vi "PCO_General.vi"() -> (0 "PCO_General":T1 {"PCO_CameraType"."wCamType" format="%x"; "PCO_CameraType"."wCamSubType" format="%x"; "PCO_CameraType"."InterfaceType" format="%x"; "dwCamHealthWarnings" format="%x"; "dwCamHealthErrors" format="%x"; "dwCamHealthStatus" format="%x"}, 1 "PCO_General_Raw":T2, 2 "Length":u16, 3 "Raw_Length":u16)   [LabVIEW 2019, in "SDK.lvlib" / "Structures.lvlib"]
doc: "Use this template to build a VI to use as a subVI."
uses:
  Structures.lvlib
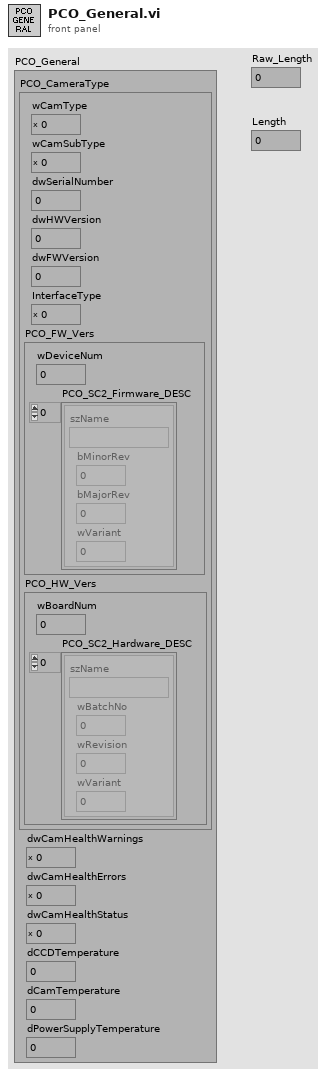
[diagram p1: front panel]
types:
  T1 = cluster{"PCO_CameraType":cluster{"wCamType":u16, "wCamSubType":u16, "dwSerialNumber":u32, "dwHWVersion":u32, "dwFWVersion":u32, "InterfaceType":u16, "PCO_FW_Vers":cluster{"wDeviceNum":u16, "PCO_SC2_Firmware_DESC":cluster{"szName":string, "bMinorRev":u8, "bMajorRev":u8, "wVariant":u16}[]}, "PCO_HW_Vers":cluster{"wBoardNum":u16, "PCO_SC2_Hardware_DESC":cluster{"szName":string, "wBatchNo":u16, "wRevision":u16, "wVariant":u16}[]}}, "dwCamHealthWarnings":u32, "dwCamHealthErrors":u32, "dwCamHealthStatus":u32, "dCCDTemperature":dbl, "dCamTemperature":dbl, "dPowerSupplyTemperature":dbl}
  T2 = cluster{"wSize":u16, "ZZwAlignDummy1":u16, "PCO_CameraType_Raw":cluster{"wSize":u16, "wCamType":u16, "wCamSubType":u16, "zzwAlignDummy1":u16, "dwSerialNumber":u32, "dwHWVersion":u32, "dwFWVersion":u32, "wInterfaceType":u16, "PCO_FW_Vers_Raw":cluster{"wDeviceNum":u16, "PCO_SC2_Firmware_DESC":cluster{"PCO_SC2_FW_Desc_Raw":cluster{"szName":cluster{u8, u8, u8, u8, u8, u8, u8, u8, u8, u8, u8, u8, u8, u8, u8, u8}, "bMinorRev":u8, "bMajorRev":u8, "wVariant":u16, "zzwDummy":cluster{u16, u16, u16, u16, u16, u16, u16, u16, u16, u16, u16, u16, u16, u16, u16, u16, u16, u16, u16, u16, u16, u16}}, "PCO_SC2_FW_Desc_Raw":cluster{"szName":cluster{u8, u8, u8, u8, u8, u8, u8, u8, u8, u8, u8, u8, u8, u8, u8, u8}, "bMinorRev":u8, "bMajorRev":u8, "wVariant":u16, "zzwDummy":cluster{u16, u16, u16, u16, u16, u16, u16, u16, u16, u16, u16, u16, u16, u16, u16, u16, u16, u16, u16, u16, u16, u16}}, "PCO_SC2_FW_Desc_Raw":cluster{"szName":cluster{u8, u8, u8, u8, u8, u8, u8, u8, u8, u8, u8, u8, u8, u8, u8, u8}, "bMinorRev":u8, "bMajorRev":u8, "wVariant":u16, "zzwDummy":cluster{u16, u16, u16, u16, u16, u16, u16, u16, u16, u16, u16, u16, u16, u16, u16, u16, u16, u16, u16, u16, u16, u16}}, "PCO_SC2_FW_Desc_Raw":cluster{"szName":cluster{u8, u8, u8, u8, u8, u8, u8, u8, u8, u8, u8, u8, u8, u8, u8, u8}, "bMinorRev":u8, "bMajorRev":u8, "wVariant":u16, "zzwDummy":cluster{u16, u16, u16, u16, u16, u16, u16, u16, u16, u16, u16, u16, u16, u16, u16, u16, u16, u16, u16, u16, u16, u16}}, "PCO_SC2_FW_Desc_Raw":cluster{"szName":cluster{u8, u8, u8, u8, u8, u8, u8, u8, u8, u8, u8, u8, u8, u8, u8, u8}, "bMinorRev":u8, "bMajorRev":u8, "wVariant":u16, "zzwDummy":cluster{u16, u16, u16, u16, u16, u16, u16, u16, u16, u16, u16, u16, u16, u16, u16, u16, u16, u16, u16, u16, u16, u16}}, "PCO_SC2_FW_Desc_Raw":cluster{"szName":cluster{u8, u8, u8, u8, u8, u8, u8, u8, u8, u8, u8, u8, u8, u8, u8, u8}, "bMinorRev":u8, "bMajorRev":u8, "wVariant":u16, "zzwDummy":cluster{u16, u16, u16, u16, u16, u16, u16, u16, u16, u16, u16, u16, u16, u16, u16, u16, u16, u16, u16, u16, u16, u16}}, "PCO_SC2_FW_Desc_Raw":cluster{"szName":cluster{u8, u8, u8, u8, u8, u8, u8, u8, u8, u8, u8, u8, u8, u8, u8, u8}, "bMinorRev":u8, "bMajorRev":u8, "wVariant":u16, "zzwDummy":cluster{u16, u16, u16, u16, u16, u16, u16, u16, u16, u16, u16, u16, u16, u16, u16, u16, u16, u16, u16, u16, u16, u16}}, "PCO_SC2_FW_Desc_Raw":cluster{"szName":cluster{u8, u8, u8, u8, u8, u8, u8, u8, u8, u8, u8, u8, u8, u8, u8, u8}, "bMinorRev":u8, "bMajorRev":u8, "wVariant":u16, "zzwDummy":cluster{u16, u16, u16, u16, u16, u16, u16, u16, u16, u16, u16, u16, u16, u16, u16, u16, u16, u16, u16, u16, u16, u16}}, "PCO_SC2_FW_Desc_Raw":cluster{"szName":cluster{u8, u8, u8, u8, u8, u8, u8, u8, u8, u8, u8, u8, u8, u8, u8, u8}, "bMinorRev":u8, "bMajorRev":u8, "wVariant":u16, "zzwDummy":cluster{u16, u16, u16, u16, u16, u16, u16, u16, u16, u16, u16, u16, u16, u16, u16, u16, u16, u16, u16, u16, u16, u16}}, "PCO_SC2_FW_Desc_Raw":cluster{"szName":cluster{u8, u8, u8, u8, u8, u8, u8, u8, u8, u8, u8, u8, u8, u8, u8, u8}, "bMinorRev":u8, "bMajorRev":u8, "wVariant":u16, "zzwDummy":cluster{u16, u16, u16, u16, u16, u16, u16, u16, u16, u16, u16, u16, u16, u16, u16, u16, u16, u16, u16, u16, u16, u16}}}}, "PCO_HW_Vers_Raw":cluster{"wBoardNum":u16, "PCO_SC2_Hardware_DESC":cluster{"PCO_SC2_HW_Desc_Raw":cluster{"szName":cluster{u8, u8, u8, u8, u8, u8, u8, u8, u8, u8, u8, u8, u8, u8, u8, u8}, "wBatchNo":u16, "wRevision":u16, "wVariant":u16, "zzwDummy":cluster{u16, u16, u16, u16, u16, u16, u16, u16, u16, u16, u16, u16, u16, u16, u16, u16, u16, u16, u16, u16}}, "PCO_SC2_HW_Desc_Raw":cluster{"szName":cluster{u8, u8, u8, u8, u8, u8, u8, u8, u8, u8, u8, u8, u8, u8, u8, u8}, "wBatchNo":u16, "wRevision":u16, "wVariant":u16, "zzwDummy":cluster{u16, u16, u16, u16, u16, u16, u16, u16, u16, u16, u16, u16, u16, u16, u16, u16, u16, u16, u16, u16}}, "PCO_SC2_HW_Desc_Raw":cluster{"szName":cluster{u8, u8, u8, u8, u8, u8, u8, u8, u8, u8, u8, u8, u8, u8, u8, u8}, "wBatchNo":u16, "wRevision":u16, "wVariant":u16, "zzwDummy":cluster{u16, u16, u16, u16, u16, u16, u16, u16, u16, u16, u16, u16, u16, u16, u16, u16, u16, u16, u16, u16}}, "PCO_SC2_HW_Desc_Raw":cluster{"szName":cluster{u8, u8, u8, u8, u8, u8, u8, u8, u8, u8, u8, u8, u8, u8, u8, u8}, "wBatchNo":u16, "wRevision":u16, "wVariant":u16, "zzwDummy":cluster{u16, u16, u16, u16, u16, u16, u16, u16, u16, u16, u16, u16, u16, u16, u16, u16, u16, u16, u16, u16}}, "PCO_SC2_HW_Desc_Raw":cluster{"szName":cluster{u8, u8, u8, u8, u8, u8, u8, u8, u8, u8, u8, u8, u8, u8, u8, u8}, "wBatchNo":u16, "wRevision":u16, "wVariant":u16, "zzwDummy":cluster{u16, u16, u16, u16, u16, u16, u16, u16, u16, u16, u16, u16, u16, u16, u16, u16, u16, u16, u16, u16}}, "PCO_SC2_HW_Desc_Raw":cluster{"szName":cluster{u8, u8, u8, u8, u8, u8, u8, u8, u8, u8, u8, u8, u8, u8, u8, u8}, "wBatchNo":u16, "wRevision":u16, "wVariant":u16, "zzwDummy":cluster{u16, u16, u16, u16, u16, u16, u16, u16, u16, u16, u16, u16, u16, u16, u16, u16, u16, u16, u16, u16}}, "PCO_SC2_HW_Desc_Raw":cluster{"szName":cluster{u8, u8, u8, u8, u8, u8, u8, u8, u8, u8, u8, u8, u8, u8, u8, u8}, "wBatchNo":u16, "wRevision":u16, "wVariant":u16, "zzwDummy":cluster{u16, u16, u16, u16, u16, u16, u16, u16, u16, u16, u16, u16, u16, u16, u16, u16, u16, u16, u16, u16}}, "PCO_SC2_HW_Desc_Raw":cluster{"szName":cluster{u8, u8, u8, u8, u8, u8, u8, u8, u8, u8, u8, u8, u8, u8, u8, u8}, "wBatchNo":u16, "wRevision":u16, "wVariant":u16, "zzwDummy":cluster{u16, u16, u16, u16, u16, u16, u16, u16, u16, u16, u16, u16, u16, u16, u16, u16, u16, u16, u16, u16}}, "PCO_SC2_HW_Desc_Raw":cluster{"szName":cluster{u8, u8, u8, u8, u8, u8, u8, u8, u8, u8, u8, u8, u8, u8, u8, u8}, "wBatchNo":u16, "wRevision":u16, "wVariant":u16, "zzwDummy":cluster{u16, u16, u16, u16, u16, u16, u16, u16, u16, u16, u16, u16, u16, u16, u16, u16, u16, u16, u16, u16}}, "PCO_SC2_HW_Desc_Raw":cluster{"szName":cluster{u8, u8, u8, u8, u8, u8, u8, u8, u8, u8, u8, u8, u8, u8, u8, u8}, "wBatchNo":u16, "wRevision":u16, "wVariant":u16, "zzwDummy":cluster{u16, u16, u16, u16, u16, u16, u16, u16, u16, u16, u16, u16, u16, u16, u16, u16, u16, u16, u16, u16}}}}, "zzWDummy":cluster{u16, u16, u16, u16, u16, u16, u16, u16, u16, u16, u16, u16, u16, u16, u16, u16, u16, u16, u16, u16, u16, u16, u16, u16, u16, u16, u16, u16, u16, u16, u16, u16, u16, u16, u16, u16, u16, u16, u16}}, "dwCamHealthWarnings":u32, "dwCamHealthErrors":u32, "dwCamHealthStatus":u32, "sCCDTemperature":i16, "sCamTemperature":i16, "sPowerSupplyTemperature":i16, "ZZwDummy":cluster{u16, u16, u16, u16, u16, u16, u16, u16, u16, u16, u16, u16, u16, u16, u16, u16, u16, u16, u16, u16, u16, u16, u16, u16, u16, u16, u16, u16, u16, u16, u16, u16, u16, u16, u16, u16, u16}}
  T3 = cluster{u16, u16, u16, u16, u16, u16, u16, u16, u16, u16, u16, u16, u16, u16, u16, u16, u16, u16, u16, u16, u16, u16, u16, u16, u16, u16, u16, u16, u16, u16, u16, u16, u16, u16, u16, u16, u16}
  T4 = cluster{"wCamType":u16, "wCamSubType":u16, "dwSerialNumber":u32, "dwHWVersion":u32, "dwFWVersion":u32, "InterfaceType":u16, "PCO_FW_Vers":cluster{"wDeviceNum":u16, "PCO_SC2_Firmware_DESC":cluster{"szName":string, "bMinorRev":u8, "bMajorRev":u8, "wVariant":u16}[]}, "PCO_HW_Vers":cluster{"wBoardNum":u16, "PCO_SC2_Hardware_DESC":cluster{"szName":string, "wBatchNo":u16, "wRevision":u16, "wVariant":u16}[]}}
  T5 = cluster{"wSize":u16, "wCamType":u16, "wCamSubType":u16, "zzwAlignDummy1":u16, "dwSerialNumber":u32, "dwHWVersion":u32, "dwFWVersion":u32, "wInterfaceType":u16, "PCO_FW_Vers_Raw":cluster{"wDeviceNum":u16, "PCO_SC2_Firmware_DESC":cluster{"PCO_SC2_FW_Desc_Raw":cluster{"szName":cluster{u8, u8, u8, u8, u8, u8, u8, u8, u8, u8, u8, u8, u8, u8, u8, u8}, "bMinorRev":u8, "bMajorRev":u8, "wVariant":u16, "zzwDummy":cluster{u16, u16, u16, u16, u16, u16, u16, u16, u16, u16, u16, u16, u16, u16, u16, u16, u16, u16, u16, u16, u16, u16}}, "PCO_SC2_FW_Desc_Raw":cluster{"szName":cluster{u8, u8, u8, u8, u8, u8, u8, u8, u8, u8, u8, u8, u8, u8, u8, u8}, "bMinorRev":u8, "bMajorRev":u8, "wVariant":u16, "zzwDummy":cluster{u16, u16, u16, u16, u16, u16, u16, u16, u16, u16, u16, u16, u16, u16, u16, u16, u16, u16, u16, u16, u16, u16}}, "PCO_SC2_FW_Desc_Raw":cluster{"szName":cluster{u8, u8, u8, u8, u8, u8, u8, u8, u8, u8, u8, u8, u8, u8, u8, u8}, "bMinorRev":u8, "bMajorRev":u8, "wVariant":u16, "zzwDummy":cluster{u16, u16, u16, u16, u16, u16, u16, u16, u16, u16, u16, u16, u16, u16, u16, u16, u16, u16, u16, u16, u16, u16}}, "PCO_SC2_FW_Desc_Raw":cluster{"szName":cluster{u8, u8, u8, u8, u8, u8, u8, u8, u8, u8, u8, u8, u8, u8, u8, u8}, "bMinorRev":u8, "bMajorRev":u8, "wVariant":u16, "zzwDummy":cluster{u16, u16, u16, u16, u16, u16, u16, u16, u16, u16, u16, u16, u16, u16, u16, u16, u16, u16, u16, u16, u16, u16}}, "PCO_SC2_FW_Desc_Raw":cluster{"szName":cluster{u8, u8, u8, u8, u8, u8, u8, u8, u8, u8, u8, u8, u8, u8, u8, u8}, "bMinorRev":u8, "bMajorRev":u8, "wVariant":u16, "zzwDummy":cluster{u16, u16, u16, u16, u16, u16, u16, u16, u16, u16, u16, u16, u16, u16, u16, u16, u16, u16, u16, u16, u16, u16}}, "PCO_SC2_FW_Desc_Raw":cluster{"szName":cluster{u8, u8, u8, u8, u8, u8, u8, u8, u8, u8, u8, u8, u8, u8, u8, u8}, "bMinorRev":u8, "bMajorRev":u8, "wVariant":u16, "zzwDummy":cluster{u16, u16, u16, u16, u16, u16, u16, u16, u16, u16, u16, u16, u16, u16, u16, u16, u16, u16, u16, u16, u16, u16}}, "PCO_SC2_FW_Desc_Raw":cluster{"szName":cluster{u8, u8, u8, u8, u8, u8, u8, u8, u8, u8, u8, u8, u8, u8, u8, u8}, "bMinorRev":u8, "bMajorRev":u8, "wVariant":u16, "zzwDummy":cluster{u16, u16, u16, u16, u16, u16, u16, u16, u16, u16, u16, u16, u16, u16, u16, u16, u16, u16, u16, u16, u16, u16}}, "PCO_SC2_FW_Desc_Raw":cluster{"szName":cluster{u8, u8, u8, u8, u8, u8, u8, u8, u8, u8, u8, u8, u8, u8, u8, u8}, "bMinorRev":u8, "bMajorRev":u8, "wVariant":u16, "zzwDummy":cluster{u16, u16, u16, u16, u16, u16, u16, u16, u16, u16, u16, u16, u16, u16, u16, u16, u16, u16, u16, u16, u16, u16}}, "PCO_SC2_FW_Desc_Raw":cluster{"szName":cluster{u8, u8, u8, u8, u8, u8, u8, u8, u8, u8, u8, u8, u8, u8, u8, u8}, "bMinorRev":u8, "bMajorRev":u8, "wVariant":u16, "zzwDummy":cluster{u16, u16, u16, u16, u16, u16, u16, u16, u16, u16, u16, u16, u16, u16, u16, u16, u16, u16, u16, u16, u16, u16}}, "PCO_SC2_FW_Desc_Raw":cluster{"szName":cluster{u8, u8, u8, u8, u8, u8, u8, u8, u8, u8, u8, u8, u8, u8, u8, u8}, "bMinorRev":u8, "bMajorRev":u8, "wVariant":u16, "zzwDummy":cluster{u16, u16, u16, u16, u16, u16, u16, u16, u16, u16, u16, u16, u16, u16, u16, u16, u16, u16, u16, u16, u16, u16}}}}, "PCO_HW_Vers_Raw":cluster{"wBoardNum":u16, "PCO_SC2_Hardware_DESC":cluster{"PCO_SC2_HW_Desc_Raw":cluster{"szName":cluster{u8, u8, u8, u8, u8, u8, u8, u8, u8, u8, u8, u8, u8, u8, u8, u8}, "wBatchNo":u16, "wRevision":u16, "wVariant":u16, "zzwDummy":cluster{u16, u16, u16, u16, u16, u16, u16, u16, u16, u16, u16, u16, u16, u16, u16, u16, u16, u16, u16, u16}}, "PCO_SC2_HW_Desc_Raw":cluster{"szName":cluster{u8, u8, u8, u8, u8, u8, u8, u8, u8, u8, u8, u8, u8, u8, u8, u8}, "wBatchNo":u16, "wRevision":u16, "wVariant":u16, "zzwDummy":cluster{u16, u16, u16, u16, u16, u16, u16, u16, u16, u16, u16, u16, u16, u16, u16, u16, u16, u16, u16, u16}}, "PCO_SC2_HW_Desc_Raw":cluster{"szName":cluster{u8, u8, u8, u8, u8, u8, u8, u8, u8, u8, u8, u8, u8, u8, u8, u8}, "wBatchNo":u16, "wRevision":u16, "wVariant":u16, "zzwDummy":cluster{u16, u16, u16, u16, u16, u16, u16, u16, u16, u16, u16, u16, u16, u16, u16, u16, u16, u16, u16, u16}}, "PCO_SC2_HW_Desc_Raw":cluster{"szName":cluster{u8, u8, u8, u8, u8, u8, u8, u8, u8, u8, u8, u8, u8, u8, u8, u8}, "wBatchNo":u16, "wRevision":u16, "wVariant":u16, "zzwDummy":cluster{u16, u16, u16, u16, u16, u16, u16, u16, u16, u16, u16, u16, u16, u16, u16, u16, u16, u16, u16, u16}}, "PCO_SC2_HW_Desc_Raw":cluster{"szName":cluster{u8, u8, u8, u8, u8, u8, u8, u8, u8, u8, u8, u8, u8, u8, u8, u8}, "wBatchNo":u16, "wRevision":u16, "wVariant":u16, "zzwDummy":cluster{u16, u16, u16, u16, u16, u16, u16, u16, u16, u16, u16, u16, u16, u16, u16, u16, u16, u16, u16, u16}}, "PCO_SC2_HW_Desc_Raw":cluster{"szName":cluster{u8, u8, u8, u8, u8, u8, u8, u8, u8, u8, u8, u8, u8, u8, u8, u8}, "wBatchNo":u16, "wRevision":u16, "wVariant":u16, "zzwDummy":cluster{u16, u16, u16, u16, u16, u16, u16, u16, u16, u16, u16, u16, u16, u16, u16, u16, u16, u16, u16, u16}}, "PCO_SC2_HW_Desc_Raw":cluster{"szName":cluster{u8, u8, u8, u8, u8, u8, u8, u8, u8, u8, u8, u8, u8, u8, u8, u8}, "wBatchNo":u16, "wRevision":u16, "wVariant":u16, "zzwDummy":cluster{u16, u16, u16, u16, u16, u16, u16, u16, u16, u16, u16, u16, u16, u16, u16, u16, u16, u16, u16, u16}}, "PCO_SC2_HW_Desc_Raw":cluster{"szName":cluster{u8, u8, u8, u8, u8, u8, u8, u8, u8, u8, u8, u8, u8, u8, u8, u8}, "wBatchNo":u16, "wRevision":u16, "wVariant":u16, "zzwDummy":cluster{u16, u16, u16, u16, u16, u16, u16, u16, u16, u16, u16, u16, u16, u16, u16, u16, u16, u16, u16, u16}}, "PCO_SC2_HW_Desc_Raw":cluster{"szName":cluster{u8, u8, u8, u8, u8, u8, u8, u8, u8, u8, u8, u8, u8, u8, u8, u8}, "wBatchNo":u16, "wRevision":u16, "wVariant":u16, "zzwDummy":cluster{u16, u16, u16, u16, u16, u16, u16, u16, u16, u16, u16, u16, u16, u16, u16, u16, u16, u16, u16, u16}}, "PCO_SC2_HW_Desc_Raw":cluster{"szName":cluster{u8, u8, u8, u8, u8, u8, u8, u8, u8, u8, u8, u8, u8, u8, u8, u8}, "wBatchNo":u16, "wRevision":u16, "wVariant":u16, "zzwDummy":cluster{u16, u16, u16, u16, u16, u16, u16, u16, u16, u16, u16, u16, u16, u16, u16, u16, u16, u16, u16, u16}}}}, "zzWDummy":cluster{u16, u16, u16, u16, u16, u16, u16, u16, u16, u16, u16, u16, u16, u16, u16, u16, u16, u16, u16, u16, u16, u16, u16, u16, u16, u16, u16, u16, u16, u16, u16, u16, u16, u16, u16, u16, u16, u16, u16}}
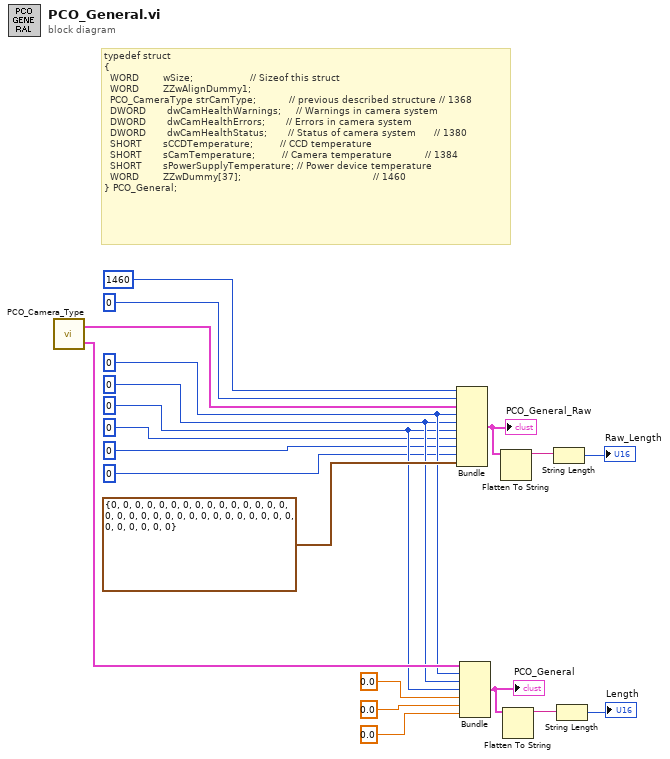
[diagram p0: block diagram]
diagram:
  w9 = u32 0 ("dwCamHealthWarnings")
  w7 = u32 0 ("dwCamHealthStatus")
  w8 = u32 0 ("dwCamHealthErrors")
  # "typedef struct\n{\n  WORD        wSize;                   // Sizeof this struct\n  WORD        ZZwAlignDummy1;\n  PCO_CameraType strCamType;           // previous described structure // 1368\n  DWORD       dwCamHealthWarnings;     // Warnings in camera system\n  DWORD       dwCamHealthErrors;       // Errors in camera system\n  DWORD       dwCamHealthStatus;       // Status of camera system      // 1380\n  SHORT       sCCDTemperature;         // CCD temperature\n  SHORT       sCamTemperature;         // Camera temperature           // 1384\n  SHORT       sPowerSupplyTemperature; // Power device temperature\n  WORD        ZZwDummy[37];                                            // 1460\n} PCO_General;"
  n1 = call "PCO_Camera_Type.vi"() -> ("PCO_CameraType"=w10:T4, "PCO_CameraType_Raw"=w12:T5)  [unwired: 4 in, 2 out]
  n2 = Bundle("wSize"=u16 1460, "ZZwAlignDummy1"=u16 0, "PCO_CameraType_Raw"=w12, "dwCamHealthWarnings"=w9, "dwCamHealthErrors"=w8, "dwCamHealthStatus"=w7, "sCCDTemperature"=i16 0, "sCamTemperature"=i16 0, "sPowerSupplyTemperature"=i16 0, "ZZwDummy"=T3 {0, 0, 0, 0, 0, 0, 0, 0, 0, 0, 0, 0, 0, 0, 0, 0, 0, 0, 0, 0, 0, 0, 0, 0, 0, 0, 0, 0, 0, 0, 0, 0, 0, 0, 0, 0, 0}) -> (w18:T2)  [unwired: 1 in]
  "PCO_General_Raw" <- w18
  n3 = Bundle("PCO_CameraType"=w10, "dwCamHealthWarnings"=w9, "dwCamHealthErrors"=w8, "dwCamHealthStatus"=w7, "dCCDTemperature"=0.0, "dCamTemperature"=0.0, "dPowerSupplyTemperature"=0.0) -> (w17:T1)  [unwired: 1 in]
  "PCO_General" <- w17
  n4 = Flatten To String(anything=w18) -> (data string=w15:string)  [unwired: 3 in, 2 out]
  n5 = Flatten To String(anything=w17) -> (data string=w16:string)  [unwired: 3 in, 2 out]
  n6 = String Length(string=w15) -> (length=→"Raw_Length":i32)
  n7 = String Length(string=w16) -> (length=→"Length":i32)
